vi "Echo_Periodic_Tasks.vi"() -> ()   [LabVIEW 2012]
panel:
  in  "Files":path[](array[path])
  in  "Read":bool
  in  "file name":path
  in  "Record":bool
  # "Array of file names\nEach file is read in order of index\nuse \"C:\\\" and \".xml\"\nExample:\n(0) \"datapath1\"   (1)   \"datapath2\"    (2)    \"datapath3\"\nshould be:\nC:\\datapath1.xml      then\nC:\\datapath2.xml      then\nC:\\datapath1.xml"
  # "Name the file that the spreadsheet data will be saved under\nuse \"C:\\\" and  \".xml\"\n\nexample:       \"datapath1\" should be \"C:\\datapath1.xml\""
  # "This VI is not automatically contained in any other VIs\n\nPlace it in Periodic Tasks, with no inputs, and outside of\nany loops.  It contains its own while loops, so putting it\nin a while loop will cause problems.\n\nIt combines  the functions of Echo Record and Echo Begin\nIn order to record data:\n -Enter the name of the file to create\n       -must be valid, try C:\\filename.xml\n -Press Record\n -Do whatever you want to record\n -Press Record again\n\nIn order to test an autonomous routine:\n -Enter the names of the files representing routines\n        -in the order that you want them to run\n -Press Read\n -Select Autonomous on driver station\n -Enable robot"
  # "Take array of names and read corresponding files\ninto the autonomous array\n\nReads the data every time it is pressed, either way"
  # "Begin and end recording:\npress once to begin, again to end"
  # "This VI contains Echo Record, which takes the Data from a Global Variable\nand writes it to a spreadsheet, and Echo Begin, which takes spreadsheet\nnames and uses them to generate and array for autonomous"
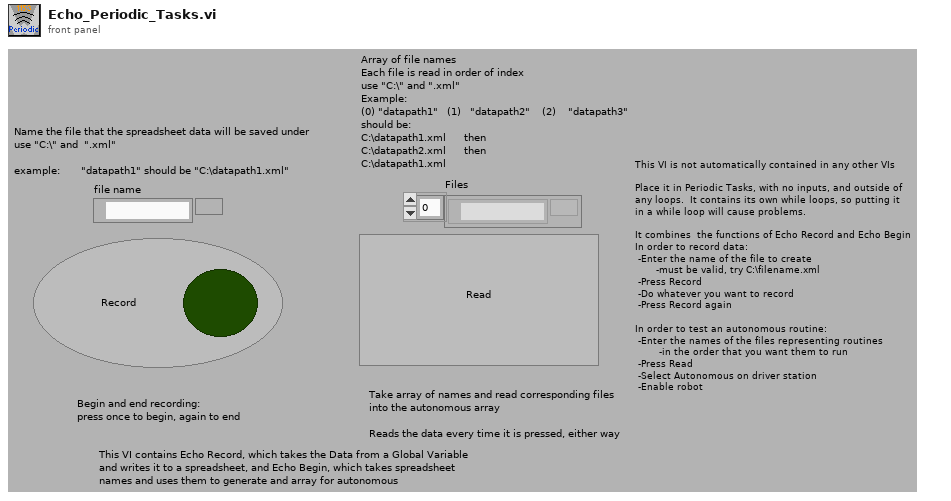
[diagram p1: front panel]
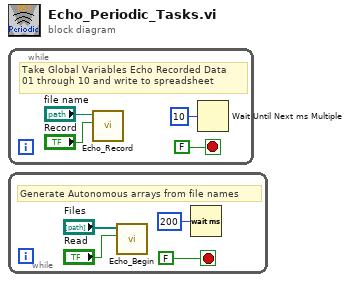
[diagram p0: block diagram]
diagram:
  n1 = while {
    stop <- FALSE stop-if-true
    # "Take Global Variables Echo Recorded Data \n01 through 10 and write to spreadsheet"
    n2 = call "Echo_Record.vi"("Record"="Record", "file name"="file name") -> ()  [unwired: 10 out]
    n3 = Wait Until Next ms Multiple(millisecond multiple=u32 10) -> ()  [unwired: 1 out]
  }
  n4 = while {
    stop <- FALSE stop-if-true
    # "Generate Autonomous arrays from file names"
    n5 = call "Echo_Begin.vi"("Read"="Read", "Files"="Files") -> ()  [unwired: 1 in, 9 out]
    n6 = Wait (ms)(milliseconds to wait=u32 200) -> ()  [unwired: 1 out]
  }
